vi "Remove response API from List.vi"(10 "API":string, 11 "output cluster in":string[](array[string])) -> (3 "output cluster out":string[](array[string]))   [LabVIEW 2020, in "Communicable State Machine.lvlib" / "BroadcastRegistry.lvclass"]
uses:
  BroadcastRegistry.lvclass
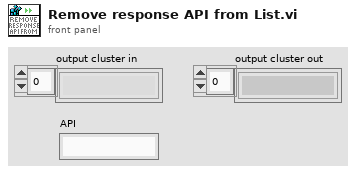
[diagram p1: front panel]
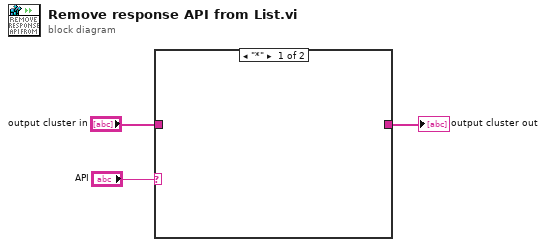
[diagram p0: block diagram]
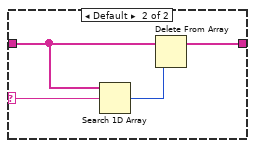
[diagram p2: hidden frame]
diagram:
  n1 = case shown="\"*\"" "API" {
    selector: "API" -> [_ w4]
    tunnel: [_ w7] -> w3
    tunnel: "output cluster in" -> [_ w6]
    frame "*" {
    }
    frame Default {
      n2 = Search 1D Array(1D array=w6, element=w4) -> (index of element=w5:i32)  [unwired: 1 in]
      n3 = Delete From Array(array=w6, index=w5) -> (array with subset deleted=w7:string[])  [unwired: 1 in, 1 out]
    }
  }
  "output cluster out" <- w3
